vi "Store Arbitrary Waveform.vi"(8 "error in (no error)":errorcluster, 9 "Waveform Generator Number (1: Waveform Generator 1)":i32(ring)=1 items=["Waveform Generator 1"=1, "Waveform Generator 2"=2], 10 "Memory Waveform Source (0: Channel 1)":i32(ring) items=["Channel 1", "Channel 2", "Channel 3", "Channel 4", "Memory Waveform 1", "Memory Waveform 2", "Function", "Math"], 11 "VISA resource name":refnum<visa-resource-name>) -> (0 "error out":errorcluster, 3 "VISA resource name out":refnum<visa-resource-name>)   [LabVIEW 2023, in "Keysight-DSQx3014T.lvlib"]
doc: "Stores the source's waveform into the arbitrary waveform memory.\n\n<b>Notes:</b>\nThis VI is not applicable for 1000 and 2000 model."
uses:
  Keysight-DSQx3014T.lvlib
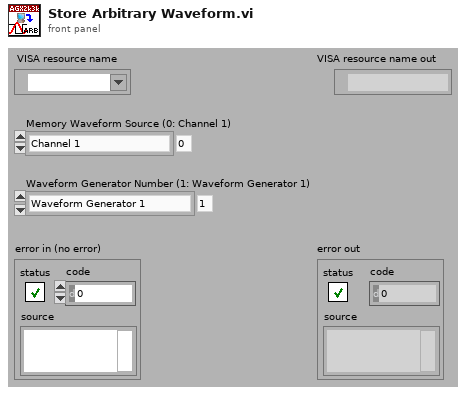
[diagram p1: front panel]
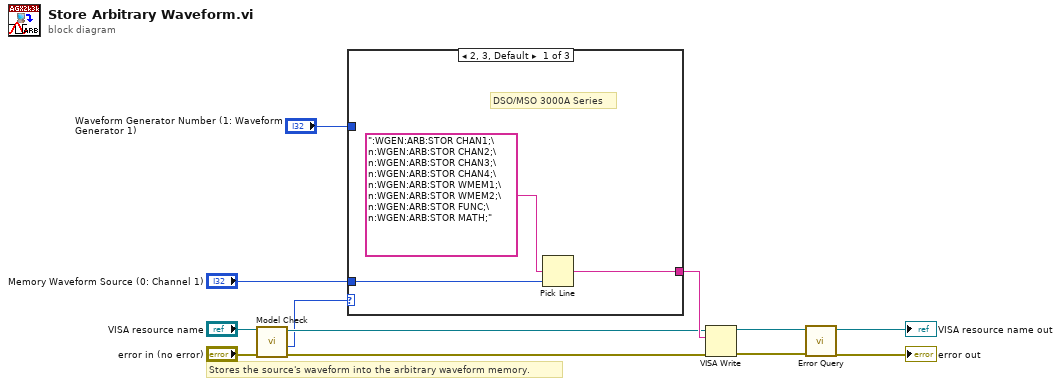
[diagram p0: block diagram]
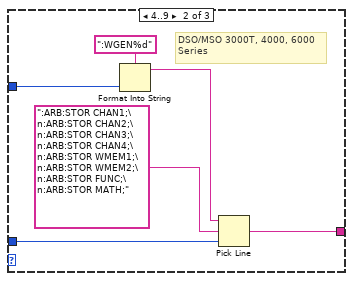
[diagram p2: hidden frame]
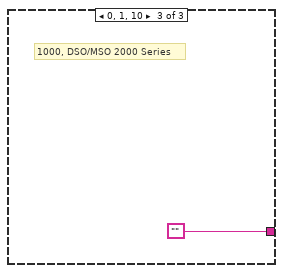
[diagram p3: hidden frame]
diagram:
  # "Stores the source's waveform into the arbitrary waveform memory."
  n1 = call "Model Check.vi"("error in (no error)"="error in (no error)", "VISA resource name"="VISA resource name") -> ("error out"=w3:errorcluster, "Model"=w1:i32, "VISA resource name out"=w4:refnum<visa-resource-name>)  [unwired: 7 out]
  n2 = case shown="2, 3, Default" w1 {
    tunnel: "Memory Waveform Source (0: Channel 1)" -> [w14 w16 _]
    tunnel: [w13 w17 ""] -> w11
    tunnel: "Waveform Generator Number (1: Waveform Generator 1)" -> [_ w20 _]
    frame 2, 3, Default {
      # "DSO/MSO 3000A Series"
      n3 = Pick Line(multi-line string=":WGEN:ARB:STOR CHAN1;\n:WGEN:ARB:STOR CHAN2;\n:WGEN:ARB:STOR CHAN3;\n:WGEN:ARB:STOR CHAN4;\n:WGEN:ARB:STOR WMEM1;\n:WGEN:ARB:STOR WMEM2;\n:WGEN:ARB:STOR FUNC;\n:WGEN:ARB:STOR MATH;", line index=w14) -> (output string=w13:string)  [unwired: 1 out]
    }
    frame 4..9 {
      # "DSO/MSO 3000T, 4000, 6000\nSeries"
      n4 = Format Into String(format string=":WGEN%d", w20) -> (resulting string=w19:string)  [unwired: 2 in, 1 out]
      n5 = Pick Line(string ("")=w19, multi-line string=":ARB:STOR CHAN1;\n:ARB:STOR CHAN2;\n:ARB:STOR CHAN3;\n:ARB:STOR CHAN4;\n:ARB:STOR WMEM1;\n:ARB:STOR WMEM2;\n:ARB:STOR FUNC;\n:ARB:STOR MATH;", line index=w16) -> (output string=w17:string)
    }
    frame 0, 1, 10 {
      # "1000, DSO/MSO 2000 Series"
    }
  }
  n6 = VISA Write(VISA resource name=w4, write buffer=w11, error in (no error)=w3) -> (VISA resource name out=w10:refnum<visa-resource-name>, error out=w9:errorcluster)  [unwired: 1 out]
  n7 = call "Error Query.vi"("error in (no error)"=w9, "VISA resource name"=w10) -> ("error out"=→"error out":errorcluster, "VISA resource name out"=→"VISA resource name out":refnum<visa-resource-name>)  [unwired: 8 out]
